vi "EZCAD.vi"() -> ()   [LabVIEW 2021]
panel:
  out "FIN":errorcluster
  in  "data in":string
  out "data out":string
  out "error out":errorcluster
  in  "stop":bool
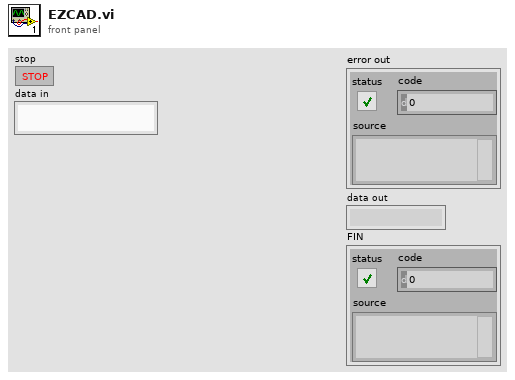
[diagram p1: front panel]
types:
  T1 = enum16{"Standard", "Buffered", "CRLF", "Immediate"}
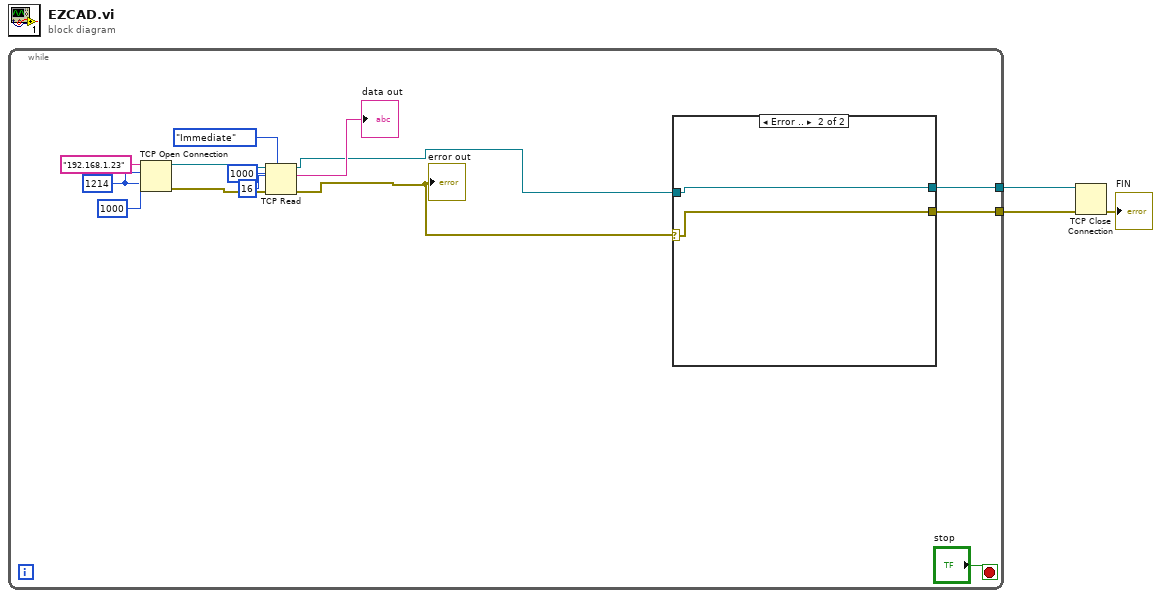
[diagram p0: block diagram]
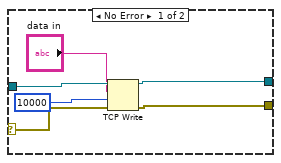
[diagram p2: hidden frame]
diagram:
  n1 = while {
    tunnel: [w8] -> w3
    tunnel: [w7] -> w2
    stop <- "stop" stop-if-true
    w6 = u16 1214 ("remote port or service name")
    n2 = TCP Open Connection(address="192.168.1.23", remote port or service name=w6, timeout ms (60000)=1000, local port=w6) -> (connection ID=w15:refnum<k5>, error out=w14:errorcluster)  [unwired: 1 in]
    n3 = TCP Read(connection ID=w15, bytes to read=16, error in (no error)=w14, 7:T1."Immediate" ("mode (standard)"), 9:1000 ("timeout ms (25000)")) -> (connection ID out=w9:refnum<k5>, data out=→"data out":string, error out=w10:errorcluster)
    "error out" <- w10
    n4 = case shown="Error .." w10 {
      selector: w10 -> [w23 w24]
      tunnel: w9 -> [w22 w25]
      tunnel: [w19 w25] -> w8
      tunnel: [w18 w24] -> w7
      frame No Error {
        n5 = TCP Write(connection ID=w22, data in="data in", error in (no error)=w23, 9:10000 ("timeout ms (25000)")) -> (connection ID out=w19:refnum<k5>, error out=w18:errorcluster)  [unwired: 1 out]
      }
      frame Error {
      }
    }
  }
  n6 = TCP Close Connection(connection ID=w3, error in (no error)=w2) -> (error out=→"FIN":errorcluster)  [unwired: 1 in, 1 out]
